vi "Global Vars.vi"() -> ()   [LabVIEW 2019]
panel:
  in  "Travel Distance":dbl=7823.0
  in  "Movement Selector":enum16{"DriveForward", "Teleop", "Nothin"}(ring)
  out "intakeReverse":bool
  out "autoDriveStatus":bool
  out "autoDrive":bool
  in  "Distance-L":dbl=-7823.0
  in  "Distance-R":dbl=7823.0
  out "fire":bool
  out "aimStatus":bool
  out "fireStatus":bool
  # "Auto Motion Magic Distance In Tics"
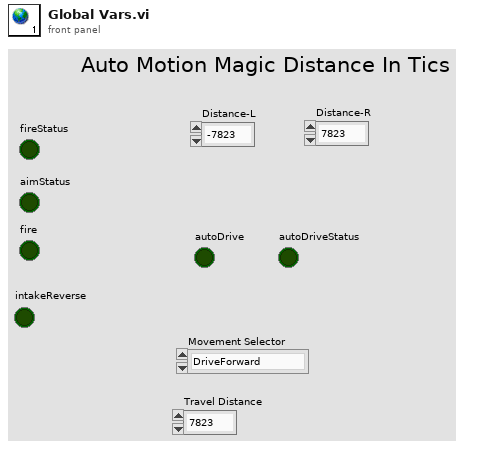
[diagram p1: front panel]
diagram:
